vi "Read Session Handle.vi"(8 "error in (no error)":errorcluster, 11 "Airmar WS in":refnum<class "Airmar WS.lvclass">) -> (0 "error out":errorcluster, 2 "hSerial":T1, 3 "Airmar WS out":refnum<class "Airmar WS.lvclass">)   [LabVIEW 2014, in "Airmar WS.lvclass"]
uses:
  Airmar WS.lvclass
  <userlib>/_Session Fwk/Session - Root.lvclass
  <userlib>/_Session Fwk/Typedefs/Session Handle.ctl
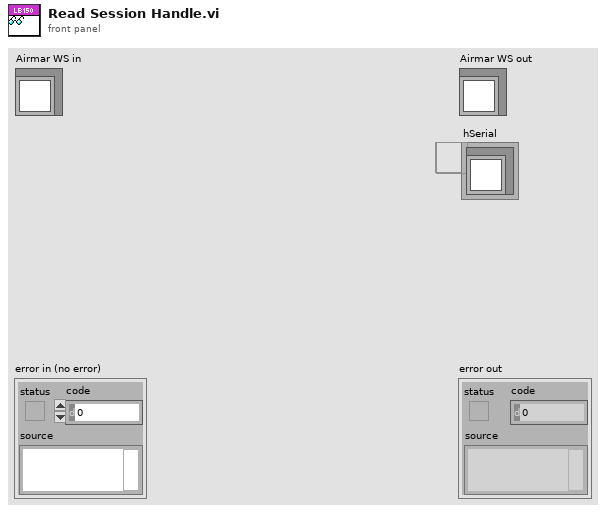
[diagram p1: front panel]
types:
  T1 = typedef "Session - Root.lvclass/Session Handle.ctl" = refnum<data-value>
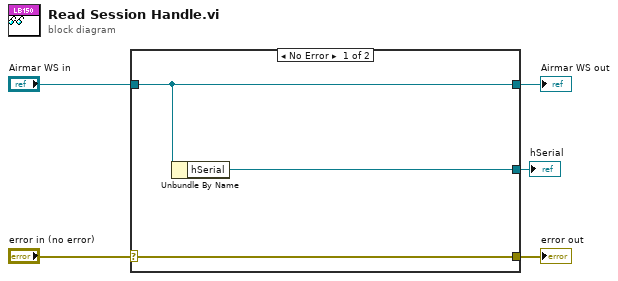
[diagram p0: block diagram]
diagram:
  n1 = case shown="No Error" "error in (no error)" {
    selector: "error in (no error)" -> [w8 w9]
    tunnel: [w8 w9] -> w4
    tunnel: [w7 w10] -> w2
    tunnel: "Airmar WS in" -> [w7 w10]
    tunnel: [w6 _] -> w1
    frame No Error {
      n2 = Unbundle By Name(w7) -> ("hSerial"=w6:T1)
    }
    frame Error {
    }
  }
  "error out" <- w4
  "Airmar WS out" <- w2
  "hSerial" <- w1
